vi "VISJS Viewer.vi"(4 "Extra Scripts":string, 5 "FileDependency out":map{path, T1}(c390), 6 "Options":string, 7 "OpenWebBrowser(False)":bool, 8 "error in":errorcluster, 9 "Embedd VISJS Librarya in HTMl File(False)":bool, 10 "HTMLFilePath":path, 11 "LibraryDependency":map{path, T3}(c390)) -> (0 "error out":errorcluster, 3 "HTMLFileContent":string)   [LabVIEW 2020, in "VISJS Viewer.lvlib"] (continued)
A,e=nb(g);if(t){var C=nb(this).constructor;A=MT(e,arguments,C)}else A=e.apply(this,arguments);return Ib(this,A)}}var RN=function(g){Cb(A,g);var t=NN(A);function A(g,e,C){return cn(this,A),t.call(this,g,e,C)}return kd(A,[{key:\"draw\",value:function(g,t,A,e,C,I){return this._drawShape(g,\"star\",4,t,A,e,C,I)}},{key:\"distanceToBorder\",value:function(g,t){return this._distanceToBorder(g,t)}}]),A}(rN);function PN(g){var t=function(){if(\"undefined\"==typeof Reflect||!MT)return!1;if(MT.sham)return!1;if(\"function\"==typeof Proxy)return!0;try{return Boolean.prototype.valueOf.call(MT(Boolean,[],(function(){}))),!0}catch(g){return!1}}();return function(){var A,e=nb(g);if(t){var C=nb(this).constructor;A=MT(e,arguments,C)}else A=e.apply(this,arguments);return Ib(this,A)}}var MN=function(g){Cb(A,g);var t=PN(A);function A(g,e,C){var I;return cn(this,A),(I=t.call(this,g,e,C))._setMargins(C),I}return kd(A,[{key:\"resize\",value:function(g,t,A){this.needsRefresh(t,A)&&(this.textSize=this.labelModule.getTextSize(g,t,A),this.width=this.textSize.width+this.margin.right+this.margin.left,this.height=this.textSize.height+this.margin.top+this.margin.bottom,this.radius=.5*this.width)}},{key:\"draw\",value:function(g,t,A,e,C,I){this.resize(g,e,C),this.left=t-this.width/2,this.top=A-this.height/2,this.enableShadow(g,I),this.labelModule.draw(g,this.left+this.textSize.width/2+this.margin.left,this.top+this.textSize.height/2+this.margin.top,e,C),this.disableShadow(g,I),this.updateBoundingBox(t,A,g,e,C)}},{key:\"distanceToBorder\",value:function(g,t){return this._distanceToBorder(g,t)}}]),A}($D);function BN(g){var t=function(){if(\"undefined\"==typeof Reflect||!MT)return!1;if(MT.sham)return!1;if(\"function\"==typeof Proxy)return!0;try{return Boolean.prototype.valueOf.call(MT(Boolean,[],(function(){}))),!0}catch(g){return!1}}();return function(){var A,e=nb(g);if(t){var C=nb(this).constructor;A=MT(e,arguments,C)}else A=e.apply(this,arguments);return Ib(this,A)}}var zN=function(g){Cb(A,g);var t=BN(A);function A(g,e,C){return cn(this,A),t.call(this,g,e,C)}return kd(A,[{key:\"draw\",value:function(g,t,A,e,C,I){return this._drawShape(g,\"triangle\",3,t,A,e,C,I)}},{key:\"distanceToBorder\",value:function(g,t){return this._distanceToBorder(g,t)}}]),A}(rN);function SN(g){var t=function(){if(\"undefined\"==typeof Reflect||!MT)return!1;if(MT.sham)return!1;if(\"function\"==typeof Proxy)return!0;try{return Boolean.prototype.valueOf.call(MT(Boolean,[],(function(){}))),!0}catch(g){return!1}}();return function(){var A,e=nb(g);if(t){var C=nb(this).constructor;A=MT(e,arguments,C)}else A=e.apply(this,arguments);return Ib(this,A)}}var ZN=function(g){Cb(A,g);var t=SN(A);function A(g,e,C){return cn(this,A),t.call(this,g,e,C)}return kd(A,[{key:\"draw\",value:function(g,t,A,e,C,I){return this._drawShape(g,\"triangleDown\",3,t,A,e,C,I)}},{key:\"distanceToBorder\",value:function(g,t){return this._distanceToBorder(g,t)}}]),A}(rN);function FN(g,t){var A=Lh(g);if(BT){var e=BT(g);t&&(e=pc(e).call(e,(function(t){return WT(g,t).enumerable}))),A.push.apply(A,e)}return A}function GN(g){for(var t=1;t<arguments.length;t++){var A,e,C=null!=arguments[t]?arguments[t]:{};t%2?Cl(A=FN(Object(C),!0)).call(A,(function(t){rb(g,t,C[t])})):HT?AD(g,HT(C)):Cl(e=FN(Object(C))).call(e,(function(t){fT(g,t,WT(C,t))}))}return g}var jN=function(){function g(t,A,e,C,I,i){cn(this,g),this.options=av(I),this.globalOptions=I,this.defaultOptions=i,this.body=A,this.edges=[],this.id=void 0,this.imagelist=e,this.grouplist=C,this.x=void 0,this.y=void 0,this.baseSize=this.options.size,this.baseFontSize=this.options.font.size,this.predefinedPosition=!1,this.selected=!1,this.hover=!1,this.labelModule=new qD(this.body,this.options,!1),this.setOptions(t)}return kd(g,[{key:\"attachEdge\",value:function(g){var t;-1===Xc(t=this.edges).call(t,g)&&this.edges.push(g)}},{key:\"detachEdge\",value:function(g){var t,A,e=Xc(t=this.edges).call(t,g);-1!=e&&Zl(A=this.edges).call(A,e,1)}},{key:\"setOptions\",value:function(t){var A=this.options.shape;if(t){if(void 0!==t.color&&(this._localColor=t.color),void 0!==t.id&&(this.id=t.id),void 0===this.id)throw new Error(\"Node must have an id\");g.checkMass(t,this.id),void 0!==t.x&&(null===t.x?(this.x=void 0,this.predefinedPosition=!1):(this.x=Gc(t.x),this.predefinedPosition=!0)),void 0!==t.y&&(null===t.y?(this.y=void 0,this.predefinedPosition=!1):(this.y=Gc(t.y),this.predefinedPosition=!0)),void 0!==t.size&&(this.baseSize=t.size),void 0!==t.value&&(t.value=SD(t.value)),g.parseOptions(this.options,t,!0,this.globalOptions,this.grouplist);var e=[t,this.options,this.defaultOptions];return this.chooser=YD(\"node\",e),this._load_images(),this.updateLabelModule(t),void 0!==t.opacity&&g.checkOpacity(t.opacity)&&(this.options.opacity=t.opacity),this.updateShape(A),void 0!==t.hidden||void 0!==t.physics}}},{key:\"_load_images\",value:function(){if((\"circularImage\"===this.options.shape||\"image\"===this.options.shape)&&void 0===this.options.image)throw new Error(\"Option image must be defined for node type '\"+this.options.shape+\"'\");if(void 0!==this.options.image){if(void 0===this.imagelist)throw new Error(\"Internal Error: No images provided\");if(\"string\"==typeof this.options.image)this.imageObj=this.imagelist.load(this.options.image,this.options.brokenImage,this.id);else{if(void 0===this.options.image.unselected)throw new Error(\"No unselected image provided\");this.imageObj=this.imagelist.load(this.options.image.unselected,this.options.brokenImage,this.id),void 0!==this.options.image.selected?this.imageObjAlt=this.imagelist.load(this.options.image.selected,this.options.brokenImage,this.id):this.imageObjAlt=void 0}}}},{key:\"getFormattingValues\",value:function(){var g={color:this.options.color.background,opacity:this.options.opacity,borderWidth:this.options.borderWidth,borderColor:this.options.color.border,size:this.options.size,borderDashes:this.options.shapeProperties.borderDashes,borderRadius:this.options.shapeProperties.borderRadius,shadow:this.options.shadow.enabled,shadowColor:this.options.shadow.color,shadowSize:this.options.shadow.size,shadowX:this.options.shadow.x,shadowY:this.options.shadow.y};if(this.selected||this.hover?!0===this.chooser?this.selected?(null!=this.options.borderWidthSelected?g.borderWidth=this.options.borderWidthSelected:g.borderWidth*=2,g.color=this.options.color.highlight.background,g.borderColor=this.options.color.highlight.border,g.shadow=this.options.shadow.enabled):this.hover&&(g.color=this.options.color.hover.background,g.borderColor=this.options.color.hover.border,g.shadow=this.options.shadow.enabled):\"function\"==typeof this.chooser&&(this.chooser(g,this.options.id,this.selected,this.hover),!1===g.shadow&&(g.shadowColor===this.options.shadow.color&&g.shadowSize===this.options.shadow.size&&g.shadowX===this.options.shadow.x&&g.shadowY===this.options.shadow.y||(g.shadow=!0))):g.shadow=this.options.shadow.enabled,void 0!==this.options.opacity){var t=this.options.opacity;g.borderColor=ev(g.borderColor,t),g.color=ev(g.color,t),g.shadowColor=ev(g.shadowColor,t)}return g}},{key:\"updateLabelModule\",value:function(t){void 0!==this.options.label&&null!==this.options.label||(this.options.label=\"\"),g.updateGroupOptions(this.options,GN(GN({},t),{},{color:t&&t.color||this._localColor||void 0}),this.grouplist);var A=this.grouplist.get(this.options.group,!1),e=[t,this.options,A,this.globalOptions,this.defaultOptions];this.labelModule.update(this.options,e),void 0!==this.labelModule.baseSize&&(this.baseFontSize=this.labelModule.baseSize)}},{key:\"updateShape\",value:function(g){if(g===this.options.shape&&this.shape)this.shape.setOptions(this.options,this.imageObj,this.imageObjAlt);else switch(this.options.shape){case\"box\":this.shape=new tN(this.options,this.body,this.labelModule);break;case\"circle\":this.shape=new IN(this.options,this.body,this.labelModule);break;case\"circularImage\":this.shape=new oN(this.options,this.body,this.labelModule,this.imageObj,this.imageObjAlt);break;case\"custom\":this.shape=new hN(this.options,this.body,this.labelModule,this.options.ctxRenderer);break;case\"database\":this.shape=new cN(this.options,this.body,this.labelModule);break;case\"diamond\":this.shape=new pN(this.options,this.body,this.labelModule);break;case\"dot\":this.shape=new vN(this.options,this.body,this.labelModule);break;case\"ellipse\":default:this.shape=new mN(this.options,this.body,this.labelModule);break;case\"icon\":this.shape=new wN(this.options,this.body,this.labelModule);break;case\"image\":this.shape=new xN(this.options,this.body,this.labelModule,this.imageObj,this.imageObjAlt);break;case\"square\":this.shape=new ON(this.options,this.body,this.labelModule);break;case\"hexagon\":this.shape=new DN(this.options,this.body,this.labelModule);break;case\"star\":this.shape=new RN(this.options,this.body,this.labelModule);break;case\"text\":this.shape=new MN(this.options,this.body,this.labelModule);break;case\"triangle\":this.shape=new zN(this.options,this.body,this.labelModule);break;case\"triangleDown\":this.shape=new ZN(this.options,this.body,this.labelModule)}this.needsRefresh()}},{key:\"select\",value:function(){this.selected=!0,this.needsRefresh()}},{key:\"unselect\",value:function(){this.selected=!1,this.needsRefresh()}},{key:\"needsRefresh\",value:function(){this.shape.refreshNeeded=!0}},{key:\"getTitle\",value:function(){return this.options.title}},{key:\"distanceToBorder\",value:function(g,t){return this.shape.distanceToBorder(g,t)}},{key:\"isFixed\",value:function(){return this.options.fixed.x&&this.options.fixed.y}},{key:\"isSelected\",value:function(){return this.selected}},{key:\"getValue\",value:function(){return this.options.value}},{key:\"getLabelSize\",value:function(){return this.labelModule.size()}},{key:\"setValueRange\",value:function(g,t,A){if(void 0!==this.options.value){var e=this.options.scaling.customScalingFunction(g,t,A,this.options.value),C=this.options.scaling.max-this.options.scaling.min;if(!0===this.options.scaling.label.enabled){var I=this.options.scaling.label.max-this.options.scaling.label.min;this.options.font.size=this.options.scaling.label.min+e*I}this.options.size=this.options.scaling.min+e*C}else this.options.size=this.baseSize,this.options.font.size=this.baseFontSize;this.updateLabelModule()}},{key:\"draw\",value:function(g){var t=this.getFormattingValues();return this.shape.draw(g,this.x,this.y,this.selected,this.hover,t)||{}}},{key:\"updateBoundingBox\",value:function(g){this.shape.updateBoundingBox(this.x,this.y,g)}},{key:\"resize\",value:function(g){var t=this.getFormattingValues();this.shape.resize(g,this.selected,this.hover,t)}},{key:\"getItemsOnPoint\",value:function(g){var t=[];return this.labelModule.visible()&&WD(this.labelModule.getSize(),g)&&t.push({nodeId:this.id,labelId:0}),WD(this.shape.boundingBox,g)&&t.push({nodeId:this.id}),t}},{key:\"isOverlappingWith\",value:function(g){return this.shape.left<g.right&&this.shape.left+this.shape.width>g.left&&this.shape.top<g.bottom&&this.shape.top+this.shape.height>g.top}},{key:\"isBoundingBoxOverlappingWith\",value:function(g){return this.shape.boundingBox.left<g.right&&this.shape.boundingBox.right>g.left&&this.shape.boundingBox.top<g.bottom&&this.shape.boundingBox.bottom>g.top}}],[{key:\"checkOpacity\",value:function(g){return 0<=g&&g<=1}},{key:\"checkCoordinateOrigin\",value:function(g){return void 0===g||\"center\"===g||\"top-left\"===g}},{key:\"updateGroupOptions\",value:function(t,A,e){var C;if(void 0!==e){var I=t.group;if(void 0!==A&&void 0!==A.group&&I!==A.group)throw new Error(\"updateGroupOptions: group values in options don't match.\");if(\"number\"==typeof I||\"string\"==typeof I&&\"\"!=I){var i=e.get(I);void 0!==i.opacity&&void 0===A.opacity&&(g.checkOpacity(i.opacity)||(console.error(\"Invalid option for node opacity. Value must be between 0 and 1, found: \"+i.opacity),i.opacity=void 0));var o=pc(C=VD(A)).call(C,(function(g){return null!=A[g]}));o.push(\"font\"),Jf(o,t,i),t.color=Iv(t.color)}}}},{key:\"parseOptions\",value:function(t,A){var e=arguments.length>2&&void 0!==arguments[2]&&arguments[2],C=arguments.length>3&&void 0!==arguments[3]?arguments[3]:{},I=arguments.length>4?arguments[4]:void 0;if(Jf([\"color\",\"fixed\",\"shadow\"],t,A,e),g.checkMass(A),void 0!==t.opacity&&(g.checkOpacity(t.opacity)||(console.error(\"Invalid option for node opacity. Value must be between 0 and 1, found: \"+t.opacity),t.opacity=void 0)),void 0!==A.opacity&&(g.checkOpacity(A.opacity)||(console.error(\"Invalid option for node opacity. Value must be between 0 and 1, found: \"+A.opacity),A.opacity=void 0)),A.shapeProperties&&!g.checkCoordinateOrigin(A.shapeProperties.coordinateOrigin)&&console.error(\"Invalid option for node coordinateOrigin, found: \"+A.shapeProperties.coordinateOrigin),dv(t,A,\"shadow\",C),void 0!==A.color&&null!==A.color){var i=Iv(A.color);Hf(t.color,i)}else!0===e&&null===A.color&&(t.color=av(C.color));void 0!==A.fixed&&null!==A.fixed&&(\"boolean\"==typeof A.fixed?(t.fixed.x=A.fixed,t.fixed.y=A.fixed):(void 0!==A.fixed.x&&\"boolean\"==typeof A.fixed.x&&(t.fixed.x=A.fixed.x),void 0!==A.fixed.y&&\"boolean\"==typeof A.fixed.y&&(t.fixed.y=A.fixed.y))),!0===e&&null===A.font&&(t.font=av(C.font)),g.updateGroupOptions(t,A,I),void 0!==A.scaling&&dv(t.scaling,A.scaling,\"label\",C.scaling)}},{key:\"checkMass\",value:function(g,t){if(void 0!==g.mass&&g.mass<=0){var A=\"\";void 0!==t&&(A=\" in node id: \"+t),console.error(\"%cNegative or zero mass disallowed\"+A+\", setting mass to 1.\",Tv),g.mass=1}}}]),g}();function LN(g,t){var A=void 0!==uh&&ln(g)||g[\"@@iterator\"];if(!A){if(Rh(g)||(A=function(g,t){var A;if(!g)return;if(\"string\"==typeof g)return VN(g,t);var e=wh(A=Object.prototype.toString.call(g)).call(A,8,-1);\"Object\"===e&&g.constructor&&(e=g.constructor.name);if(\"Map\"===e||\"Set\"===e)return Uo(g);if(\"Arguments\"===e||/^(?:Ui|I)nt(?:8|16|32)(?:Clamped)?Array$/.test(e))return VN(g,t)}(g))||t&&g&&\"number\"==typeof g.length){A&&(g=A);var e=0,C=function(){};return{s:C,n:function(){return e>=g.length?{done:!0}:{done:!1,value:g[e++]}},e:function(g){throw g},f:C}}throw new TypeError(\"Invalid attempt to iterate non-iterable instance.\\nIn order to be iterable, non-array objects must have a [Symbol.iterator]() method.\")}var I,i=!0,o=!1;return{s:function(){A=A.call(g)},n:function(){var g=A.next();return i=g.done,g},e:function(g){o=!0,I=g},f:function(){try{i||null==A.return||A.return()}finally{if(o)throw I}}}}function VN(g,t){(null==t||t>g.length)&&(t=g.length);for(var A=0,e=new Array(t);A<t;A++)e[A]=g[A];return e}var YN=function(){function g(t,A,e,C){var I,i=this;if(cn(this,g),this.body=t,this.images=A,this.groups=e,this.layoutEngine=C,this.body.functions.createNode=je(I=this.create).call(I,this),this.nodesListeners={add:function(g,t){i.add(t.items)},update:function(g,t){i.update(t.items,t.data,t.oldData)},remove:function(g,t){i.remove(t.items)}},this.defaultOptions={borderWidth:1,borderWidthSelected:void 0,brokenImage:void 0,color:{border:\"#2B7CE9\",background:\"#97C2FC\",highlight:{border:\"#2B7CE9\",background:\"#D2E5FF\"},hover:{border:\"#2B7CE9\",background:\"#D2E5FF\"}},opacity:void 0,fixed:{x:!1,y:!1},font:{color:\"#343434\",size:14,face:\"arial\",background:\"none\",strokeWidth:0,strokeColor:\"#ffffff\",align:\"center\",vadjust:0,multi:!1,bold:{mod:\"bold\"},boldital:{mod:\"bold italic\"},ital:{mod:\"italic\"},mono:{mod:\"\",size:15,face:\"monospace\",vadjust:2}},group:void 0,hidden:!1,icon:{face:\"FontAwesome\",code:void 0,size:50,color:\"#2B7CE9\"},image:void 0,imagePadding:{top:0,right:0,bottom:0,left:0},label:void 0,labelHighlightBold:!0,level:void 0,margin:{top:5,right:5,bottom:5,left:5},mass:1,physics:!0,scaling:{min:10,max:30,label:{enabled:!1,min:14,max:30,maxVisible:30,drawThreshold:5},customScalingFunction:function(g,t,A,e){if(t===g)return.5;var C=1/(t-g);return Math.max(0,(e-g)*C)}},shadow:{enabled:!1,color:\"rgba(0,0,0,0.5)\",size:10,x:5,y:5},shape:\"ellipse\",shapeProperties:{borderDashes:!1,borderRadius:6,interpolation:!0,useImageSize:!1,useBorderWithImage:!1,coordinateOrigin:\"center\"},size:25,title:void 0,value:void 0,x:void 0,y:void 0},this.defaultOptions.mass<=0)throw\"Internal error: mass in defaultOptions of NodesHandler may not be zero or negative\";this.options=av(this.defaultOptions),this.bindEventListeners()}return kd(g,[{key:\"bindEventListeners\",value:function(){var g,t,A=this;this.body.emitter.on(\"refreshNodes\",je(g=this.refresh).call(g,this)),this.body.emitter.on(\"refresh\",je(t=this.refresh).call(t,this)),this.body.emitter.on(\"destroy\",(function(){tv(A.nodesListeners,(function(g,t){A.body.data.nodes&&A.body.data.nodes.off(t,g)})),delete A.body.functions.createNode,delete A.nodesListeners.add,delete A.nodesListeners.update,delete A.nodesListeners.remove,delete A.nodesListeners}))}},{key:\"setOptions\",value:function(g){if(void 0!==g){if(jN.parseOptions(this.options,g),void 0!==g.opacity&&(jm(g.opacity)||!Ym(g.opacity)||g.opacity<0||g.opacity>1?console.error(\"Invalid option for node opacity. Value must be between 0 and 1, found: \"+g.opacity):this.options.opacity=g.opacity),void 0!==g.shape)for(var t in this.body.nodes)Object.prototype.hasOwnProperty.call(this.body.nodes,t)&&this.body.nodes[t].updateShape();if(void 0!==g.font||void 0!==g.widthConstraint||void 0!==g.heightConstraint)for(var A=0,e=Lh(this.body.nodes);A<e.length;A++){var C=e[A];this.body.nodes[C].updateLabelModule(),this.body.nodes[C].needsRefresh()}if(void 0!==g.size)for(var I in this.body.nodes)Object.prototype.hasOwnProperty.call(this.body.nodes,I)&&this.body.nodes[I].needsRefresh();void 0===g.hidden&&void 0===g.physics||this.body.emitter.emit(\"_dataChanged\")}}},{key:\"setData\",value:function(g){var t=arguments.length>1&&void 0!==arguments[1]&&arguments[1],A=this.body.data.nodes;if(kD(\"id\",g))this.body.data.nodes=g;else if(Rh(g))this.body.data.nodes=new mD,this.body.data.nodes.add(g);else{if(g)throw new TypeError(\"Array or DataSet expected\");this.body.data.nodes=new mD}if(A&&tv(this.nodesListeners,(function(g,t){A.off(t,g)})),this.body.nodes={},this.body.data.nodes){var e=this;tv(this.nodesListeners,(function(g,t){e.body.data.nodes.on(t,g)}));var C=this.body.data.nodes.getIds();this.add(C,!0)}!1===t&&this.body.emitter.emit(\"_dataChanged\")}},{key:\"add\",value:function(g){for(var t,A=arguments.length>1&&void 0!==arguments[1]&&arguments[1],e=[],C=0;C<g.length;C++){t=g[C];var I=this.body.data.nodes.get(t),i=this.create(I);e.push(i),this.body.nodes[t]=i}this.layoutEngine.positionInitially(e),!1===A&&this.body.emitter.emit(\"_dataChanged\")}},{key:\"update\",value:function(g,t,A){for(var e=this.body.nodes,C=!1,I=0;I<g.length;I++){var i=g[I],o=e[i],n=t[I];void 0!==o?o.setOptions(n)&&(C=!0):(C=!0,o=this.create(n),e[i]=o)}C||void 0===A||(C=Xm(t).call(t,(function(g,t){var e=A[t];return e&&e.level!==g.level}))),!0===C?this.body.emitter.emit(\"_dataChanged\"):this.body.emitter.emit(\"_dataUpdated\")}},{key:\"remove\",value:function(g){for(var t=this.body.nodes,A=0;A<g.length;A++){delete t[g[A]]}this.body.emitter.emit(\"_dataChanged\")}},{key:\"create\",value:function(g){return new(arguments.length>1&&void 0!==arguments[1]?arguments[1]:jN)(g,this.body,this.images,this.groups,this.options,this.defaultOptions)}},{key:\"refresh\",value:function(){var g=this,t=arguments.length>0&&void 0!==arguments[0]&&arguments[0];tv(this.body.nodes,(function(A,e){var C=g.body.data.nodes.get(e);void 0!==C&&(!0===t&&A.setOptions({x:null,y:null}),A.setOptions({fixed:!1}),A.setOptions(C))}))}},{key:\"getPositions\",value:function(g){var t={};if(void 0!==g){if(!0===Rh(g)){for(var A=0;A<g.length;A++)if(void 0!==this.body.nodes[g[A]]){var e=this.body.nodes[g[A]];t[g[A]]={x:Math.round(e.x),y:Math.round(e.y)}}}else if(void 0!==this.body.nodes[g]){var C=this.body.nodes[g];t[g]={x:Math.round(C.x),y:Math.round(C.y)}}}else for(var I=0;I<this.body.nodeIndices.length;I++){var i=this.body.nodes[this.body.nodeIndices[I]];t[this.body.nodeIndices[I]]={x:Math.round(i.x),y:Math.round(i.y)}}return 
